vi "Dashboard Main.vi"() -> ()   [LabVIEW 2012]
uses:
  <vilib>/event_ctls.llb/eventvkey.ctl
  <vilib>/Utility/config.llb/Read Key (String).vi
  <vilib>/Utility/config.llb/Read Key (I32).vi
  <vilib>/Utility/config.llb/Write Key (String).vi
  <vilib>/Utility/config.llb/Write Key (I32).vi
  <vilib>/Utility/config.llb/NI_LVConfig.lvlib
panel:
  out "Mode":T1(ring)=enum."Auto Disabled"
  in  "Viewer":enum32{"Camera Image", "Variables"}(tab)
  out "Mbps":dbl format="%#.1g"
  in  "Enable":bool
  in  "DB Camera Config":bool
  out "Mbps":bool
  out "fps":dbl format="%#.1g"
  out "Image Error Message":string="Timeout in Camera Communications"
  out "Camera Image":T2(plugin-control)
  out "Camera Image 2":T2(plugin-control)
  in  "Camera Settings":T3={"Frame Rate"=15, "Compression"=30, "Size"=1} {"Frame Rate" scale=1.0..30.0; "Size" items=["640x480", "320x240", "160x120"]}
  out "Camera IP 2":string
  out "Camera IP":string
  out "fps 2":dbl format="%#.1g"
  out "Mbps 2":dbl format="%#.1g"
  in  "Enable 2":bool
  in  "FR":i32=15
  out "Tree":string(tree)
  in  "Dashboard Tab":enum32{"Operation", "Test", "Checklist"}(tab)
  in  "AutonRefresh":bool
  out "Autons":string[](array[string])
  in  "Selector":bool[](array[boolean])
  in  "Slider":dbl(slide) scale=0.0..100.0 scale format="%#_3g"
  in  "On/Off":bool caption="Solenoid"
  in  "Test Name":u16(ring) items=["Select the test to run...", "Example Test", "-------------------------------", "List of tests is built in robot code.", "Replace with your own automated tests."]
  in  "Test Tree":string(tree)
  in  "Motor":cluster{"Value":dbl, "Enable":bool} {"Value" scale=-1.0..1.0 scale format="%#_3g"}
  out "Progress":T4 {"Test Progress" scale=0.0..100.0}
  in  "Rev/Fwd":cluster{"Forward":bool, "Reverse":bool}
  in  "Ring":u16(ring) items=["Auto", "Fixed indoor", "Fixed outdoor 1", "Fixed outdoor 2", "Fixed fluorescent 1", "Fixed fluorescent 2", "Hold current"]
  in  "Listbox":i32(listbox)
  out "Robot IP":string
  out "Battery Value":dbl(slide) scale=0.0..14.0 scale format="%#_2e"
  out "Battery":sgl(graph)
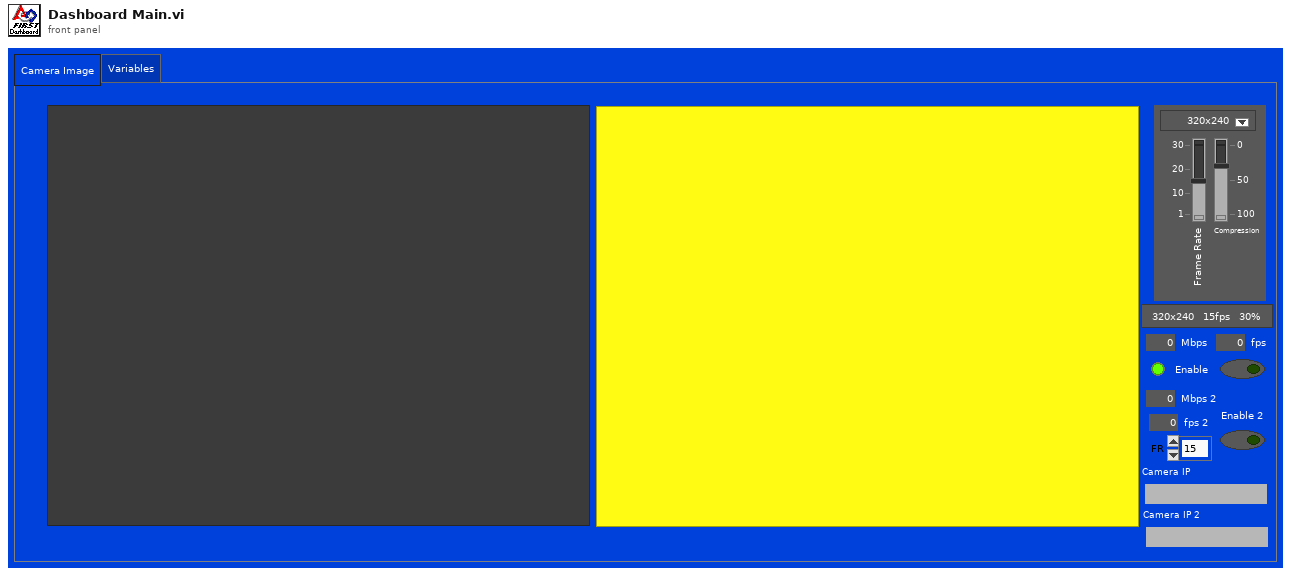
[diagram p1: front panel]
types:
  T1 = enum8{"Tele-Op Disabled", "Tele-Op Enabled", "Auto Disabled", "Auto Enabled", "Test Disabled", "Test Enabled", ""}
  T2 = typedef "IMAQ Image.ctl" = refnum<image>
  T3 = cluster{"Frame Rate":i32, "Compression":i32, "Size":u16}
  T4 = cluster{"Test Progress":u8, "Test Progress Text":string}
  T5 = typedef "Image Type" = u32
  T6 = cluster{"Competition mode":bool, "Robot Link":bool, "Autonomous":bool, "Enabled":bool, "E-Stop":bool, "Simulated":bool, "TestMode":bool, "Docked Window":bool}
  T7 = typedef "LVRectTypeDef.ctl" = cluster{"Left":i16, "Top":i16, "Right":i16, "Bottom":i16}
  T8 = typedef "NI_LVConfig.lvlib/Config Data RefNum.ctl" = refnum<k1>
  T9 = typedef "eventvkey.ctl" = enum16{"ASCII", "Enter", "Return", "Shift", "Ctrl", "Alt", "Cmd", "Opt", "Caps", "NumLock", "Clear", "Break", "Up", "Down", "Left", "Right", "Insert", "Delete", "Home", "End", "PageUp", "PageDown", "Escape", "Help", "Pause", "ScrollLock", "F1", "F2", "F3", "F4", "F5", "F6", "F7", "F8", "F9", "F10", "F11", "F12", "F13", "F14", "F15", "F16", "F17", "F18", "F19", "F20", "F21", "F22", "F23", "F24", "Play", "VolumeUp", "VolumeDown", "Mute", "Two Byte Char"}
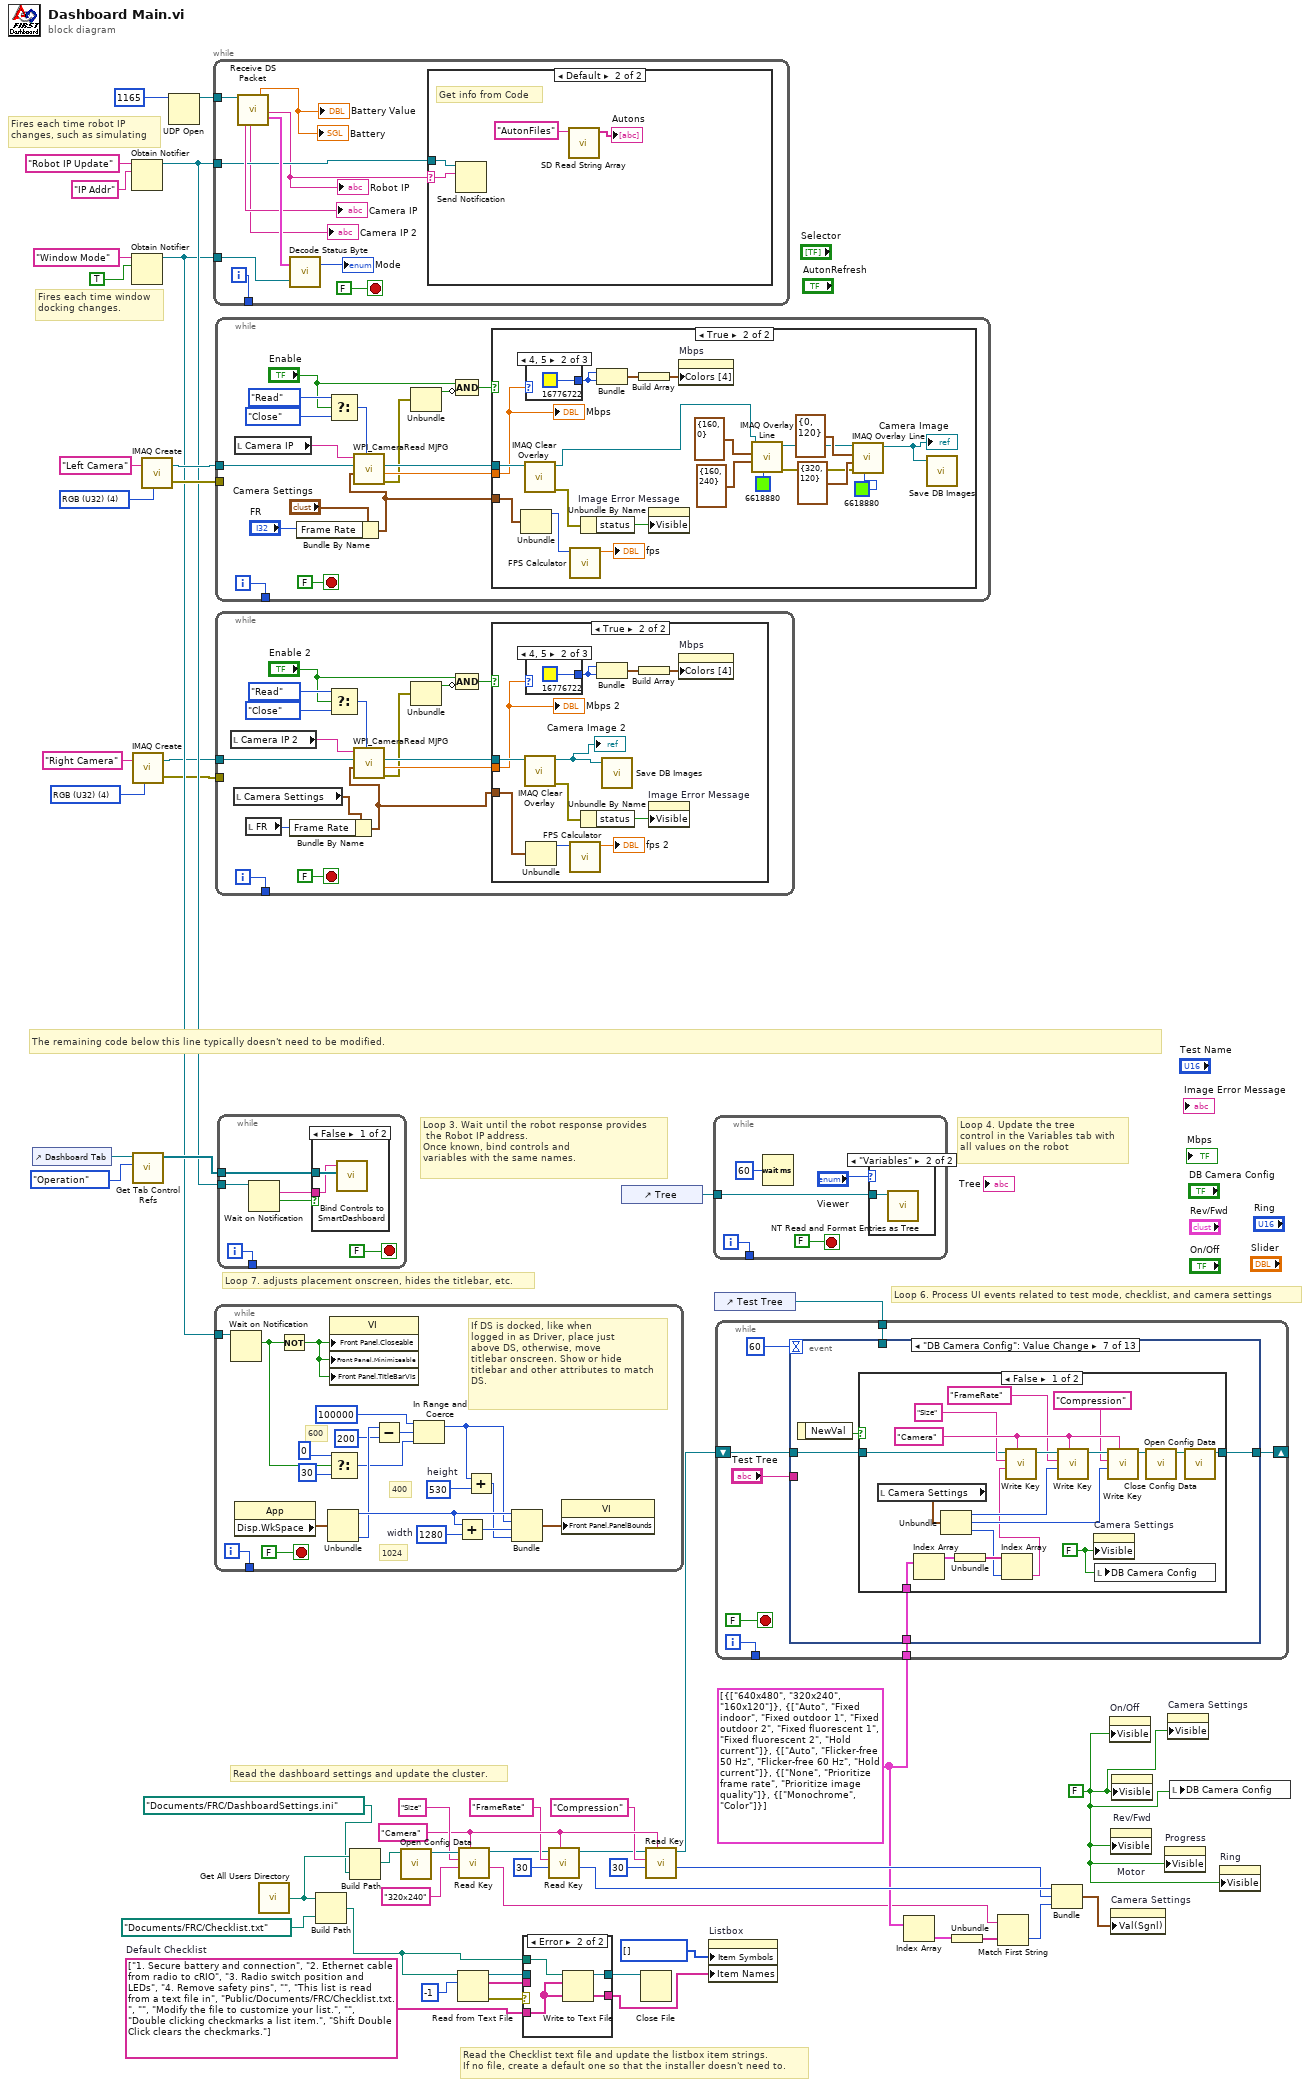
[diagram p0: block diagram]
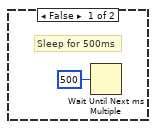
[diagram p2: hidden frame]
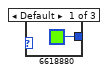
[diagram p3: hidden frame]
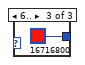
[diagram p4: hidden frame]
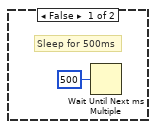
[diagram p6: hidden frame]
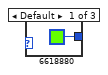
[diagram p7: hidden frame]
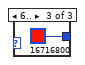
[diagram p8: hidden frame]
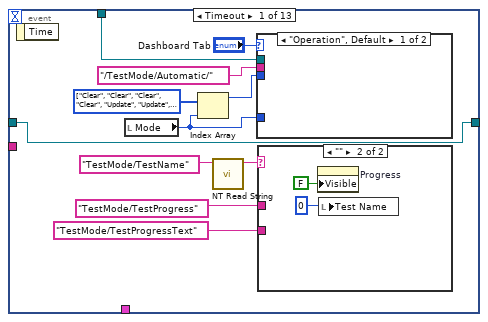
[diagram p10: hidden frame]
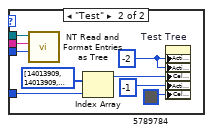
[diagram p11: hidden frame]
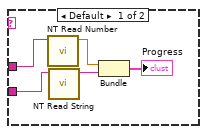
[diagram p12: hidden frame]
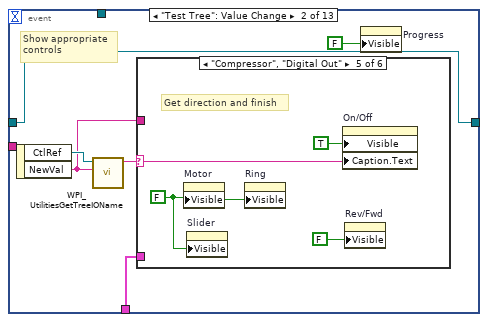
[diagram p13: hidden frame]
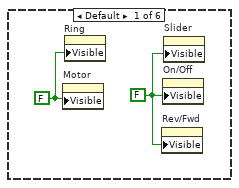
[diagram p14: hidden frame]
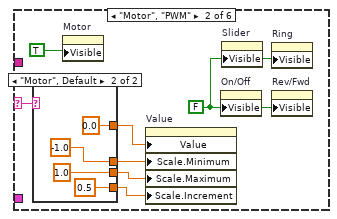
[diagram p15: hidden frame]
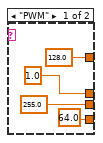
[diagram p16: hidden frame]
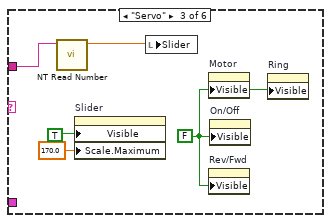
[diagram p17: hidden frame]
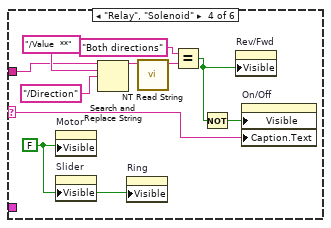
[diagram p18: hidden frame]
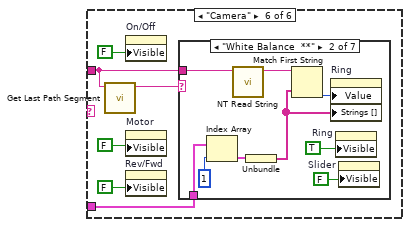
[diagram p19: hidden frame]
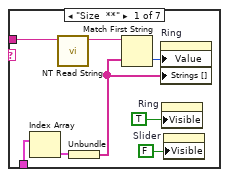
[diagram p20: hidden frame]
diagram:
  w3 = T5 4 items=["Grayscale (U8)", "Grayscale (I16)", "Grayscale (SGL)", "Complex (CSG)", "RGB (U32)", "HSL (U32)", "RGB (U64)"] ("Image Type")
  w25 = "Camera"
  w17 = cluster{string[]}[] [{["640x480", "320x240", "160x120"]}, {["Auto", "Fixed indoor", "Fixed outdoor 1", "Fixed outdoor 2", "Fixed fluorescent 1", "Fixed fluorescent 2", "Hold current"]}, {["Auto", "Flicker-free 50 Hz", "Flicker-free 60 Hz", "Hold current"]}, {["None", "Prioritize frame rate", "Prioritize image quality"]}, {["Monochrome", "Color"]}]
  w33 = string[] ["1. Secure battery and connection", "2. Ethernet cable from radio to cRIO", "3. Radio switch position and LEDs", "4. Remove safety pins", "", "This list is read from a text file in", "Public/Documents/FRC/Checklist.txt.", "", "Modify the file to customize your list.", "", "Double clicking checkmarks a list item.", "Shift Double Click clears the checkmarks."]  # Default Checklist
  w31 = FALSE ("Visible")
  w52 = T5 4 items=["Grayscale (U8)", "Grayscale (I16)", "Grayscale (SGL)", "Complex (CSG)", "RGB (U32)", "HSL (U32)", "RGB (U64)"] ("Image Type")
  # "Fires each time robot IP\nchanges, such as simulating"
  # "Fires each time window\ndocking changes."
  # "Read the Checklist text file and update the listbox item strings.\nIf no file, create a default one so that the installer doesn't need to."
  # "The remaining code below this line typically doesn't need to be modified."
  # "Loop 6. Process UI events related to test mode, checklist, and camera settings"
  # "Read the dashboard settings and update the cluster."
  # "Loop 4. Update the tree\ncontrol in the Variables tab with\nall values on the robot"
  # "Loop 3. Wait until the robot response provides\n the Robot IP address.\nOnce known, bind controls and\nvariables with the same names."
  # "Loop 7. adjusts placement onscreen, hides the titlebar, etc."
  n1 = control-ref of="Dashboard Tab"() -> (w47:refnum<vi>)
  n2 = Obtain Notifier(name (unnamed)="Robot IP Update", notification data type="IP Addr" ("name (unnamed)")) -> (notifier out=w44:refnum<notifier>)  [unwired: 2 in, 2 out]
  n3 = Obtain Notifier(name (unnamed)="Window Mode", notification data type=TRUE) -> (notifier out=w37:refnum<notifier>)  [unwired: 2 in, 2 out]
  n4 = call "IMAQ Create"("Image Name"="Right Camera", "Image Type"=w3) -> ("New Image"=w2:T2, "error out"=w1:errorcluster)  [unwired: 2 in, 1 out]
  n5 = call <vilib>:"Get Tab Control Refs.vi"("Page Index"=enum32{"Operation", "Test"}."Operation" ("Dashboard Tab"), "TabControl in"=w47) -> ("ControlsOnPage"=w48:refnum<vi>[])  [unwired: 9 in]
  n6 = call "IMAQ Create"("Image Name"="Left Camera", "Image Type"=w52) -> ("New Image"=w50:T2, "error out"=w49:errorcluster)  [unwired: 2 in, 1 out]
  n7 = UDP Open(11:u16 1165 ("port")) -> (port=w53:refnum<k16>)  [unwired: 2 in, 4 out]
  n8 = while {
    tunnel: w53 -> [w63]
    tunnel: w44 -> [w57]
    tunnel: w37 -> [w61]
    tunnel: [w58] -> _
    i -> [w58]
    stop <- FALSE stop-if-true
    n9 = call "Receive DS Packet.vi"("Recv Socket"=w63) -> ("Camera IP Address"=→"Camera IP":string, "Camera IP Address 2"=→"Camera IP 2":string, "Battery"=→"Battery" →"Battery Value":sgl, "Robot IP Address"=w56:string, "Status"=w64:T6)  [unwired: 8 in, 6 out]
    "Robot IP" <- w56
    n10 = call "Decode Status Byte.vi"("Window Mode Notifier"=w61, "Status"=w64) -> ("Mode"=→"Mode":T1)  [unwired: 1 out]
    n11 = case shown="Default" w56 {
      selector: w56 -> [_ w68]
      tunnel: w57 -> [_ w69]
      frame "0.0.0.0" {
        # "Robot not responding, don't poll the variables"
      }
      frame Default {
        # "Get info from Code"
        n12 = Send Notification(notification=w68, notifier=w69) -> ()  [unwired: 1 in, 2 out]
        n13 = call <vilib>:"SD Read String Array.vi"("Name"="AutonFiles") -> ("String Array"=→"Autons":string[])  [unwired: 9 in, 1 out]
      }
    }
  }
  n14 = while {
    tunnel: w37 -> [w88]
    tunnel: [w86] -> _
    i -> [w86]
    stop <- FALSE stop-if-true
    w78 = 1280  # width
    w81 = 530  # height
    # "600"
    # "1024"
    # "400"
    # "If DS is docked, like when\nlogged in as Driver, place just\nabove DS, otherwise, move\ntitlebar onscreen. Show or hide\ntitlebar and other attributes to match\nDS."
    n15 = Wait on Notification(notifier=w88) -> (notification=w73:bool)  [unwired: 3 in, 3 out]
    n16 = property class="App"() -> ("Disp.WkSpace"=w84:T7)  [unwired: 2 in, 2 out]
    n17 = Not(x=w73) -> (.not. x?=w87:bool)
    n18 = Unbundle(w84) -> ("Left"=w82:i16, "Bottom"=w79:i16)  [unwired: 2 out]
    n19 = Select(t=0, s=w73, f=30) -> (s? t:f=w72:i32)
    n20 = property class="VI"("Front Panel.Closeable"=w87, "Front Panel.Minimizeable"=w87, "Front Panel.TitleBarVis"=w87) -> ()  [unwired: 2 in, 2 out]
    n21 = Subtract(x=w79, y=200) -> (x-y=w76:i32)
    n22 = In Range and Coerce(upper limit=100000, x=w76, lower limit=w72) -> (coerced(x)=w70:i32)  [unwired: 1 out]
    n23 = Add(x=w82, y=w78) -> (x+y=w83:i32)
    n24 = Add(x=w70, y=w81) -> (x+y=w80:i32)
    n25 = Bundle("Left"=w82, w70, w83, w80) -> (w85:cluster{"Left":i16, i32, i32, i32})  [unwired: 1 out]
    n26 = property class="VI"("Front Panel.PanelBounds"=w85) -> ()  [unwired: 2 in, 2 out]
  }
  n27 = while {
    tunnel: w50 -> [w102]
    tunnel: w49 -> [_]
    tunnel: [w104] -> _
    i -> [w104]
    stop <- FALSE stop-if-true
    n28 = local read "Camera IP"() -> (w103:string)
    n29 = Bundle By Name(cluster="Camera Settings", "Frame Rate"="FR") -> (w90:T3)
    n30 = Select(t=enum16{"Read", "Reopen", "Close"}."Read" ("Operation"), s="Enable", f=enum16{"Read", "Reopen", "Close"}."Close" ("Operation")) -> (s? t:f=w97:enum16{"Read", "Reopen", "Close"})
    n31 = call <vilib>:"WPI_CameraRead MJPG.vi"("Operation"=w97, "Camera Settings"=w90, "Image"=w102, "address"=w103) -> ("error out"=w96:errorcluster, "Bandwidth (kbps)"=w100:dbl, "Image Out"=w101:T2)  [unwired: 5 in]
    n32 = Unbundle(w96) -> ("status"=w94:bool)  [unwired: 2 out]
    n33 = Compound Arithmetic op=AND("Enable", invert w94) -> (w93:bool)
    n34 = case shown="True" w93 {
      tunnel: w90 -> [_ w118]
      tunnel: w101 -> [_ w121]
      tunnel: w100 -> [_ w120]
      frame False {
        # "Sleep for 500ms"
        n35 = Wait Until Next ms Multiple(millisecond multiple=u32 500) -> ()  [unwired: 1 out]
      }
      frame True {
        n36 = Unbundle(w118) -> ("Frame Rate"=w108:i32)  [unwired: 2 out]
        n37 = call "IMAQ Clear Overlay"("Image"=w121) -> ("error out"=w125:errorcluster, "Image Out"=w110:T2)  [unwired: 2 in, 7 out]
        n38 = case shown="4, 5" w120 {
          tunnel: [u32 6618880 ("Color Box") u32 16776722 ("Color Box") u32 16716800 ("Color Box")] -> w122
          frame Default {
          }
          frame 4, 5 {
          }
          frame 6.. {
          }
        }
        n39 = call "FPS Calculator.vi"("Average Count"=w108) -> ("fps"=→"fps":dbl)  [unwired: 10 in]
        n40 = Unbundle By Name(w125) -> ("status"=w126:bool)
        n41 = Bundle("Color Box"=w122, "Color Box"=w122) -> (w124:cluster{"Color Box":u32, "Color Box":u32})  [unwired: 1 out]
        n42 = Build Array(w124) -> (w123:cluster{"Color Box":u32, "Color Box":u32}[])
        n43 = property on="Image Error Message" class="Str"("Visible"=w126) -> ()  [unwired: 2 in, 2 out]
        n44 = property on="Mbps" class="Bool (strict)"("Colors [4]"=w123) -> ()  [unwired: 2 in, 2 out]
        n45 = call "IMAQ Overlay Line"("Color"=u32 6618880, "End Point"=cluster{"X":i32, "Y":i32} {"X"=160, "Y"=240}, "Start Point"=cluster{"X":i32, "Y":i32} {"X"=160, "Y"=0}, "Image"=w110) -> ("error out"=w115:errorcluster, "Image Out"=w114:T2)  [unwired: 6 in]
        n46 = call "IMAQ Overlay Line"("Color"=u32 6618880, "error in (no error)"=w115, "End Point"=cluster{"X":i32, "Y":i32} {"X"=320, "Y"=120}, "Start Point"=cluster{"X":i32, "Y":i32} {"X"=0, "Y"=120}, "Image"=w114) -> ("Image Out"=w109:T2)  [unwired: 5 in, 1 out]
        "Camera Image" <- w109
        n47 = call "Save DB Images.vi"("Image"=w109) -> ()  [unwired: 2 in, 1 out]
        "Mbps" <- w120
      }
    }
  }
  n48 = while {
    tunnel: w2 -> [w142]
    tunnel: [w144] -> _
    tunnel: w1 -> [_]
    i -> [w144]
    stop <- FALSE stop-if-true
    n49 = local read "Camera IP 2"() -> (w143:string)
    n50 = local read "Camera Settings"() -> (w131:T3)
    n51 = local read "FR"() -> (w132:i32)
    n52 = Bundle By Name(cluster=w131, "Frame Rate"=w132) -> (w130:T3)
    n53 = Select(t=enum16{"Read", "Reopen", "Close"}."Read" ("Operation"), s="Enable 2", f=enum16{"Read", "Reopen", "Close"}."Close" ("Operation")) -> (s? t:f=w137:enum16{"Read", "Reopen", "Close"})
    n54 = call <vilib>:"WPI_CameraRead MJPG.vi"("Operation"=w137, "Camera Settings"=w130, "Image"=w142, "address"=w143) -> ("error out"=w136:errorcluster, "Bandwidth (kbps)"=w140:dbl, "Image Out"=w141:T2)  [unwired: 5 in]
    n55 = Unbundle(w136) -> ("status"=w134:bool)  [unwired: 2 out]
    n56 = Compound Arithmetic op=AND("Enable 2", invert w134) -> (w133:bool)
    n57 = case shown="True" w133 {
      tunnel: w130 -> [_ w149]
      tunnel: w141 -> [_ w152]
      tunnel: w140 -> [_ w151]
      frame False {
        # "Sleep for 500ms"
        n58 = Wait Until Next ms Multiple(millisecond multiple=u32 500) -> ()  [unwired: 1 out]
      }
      frame True {
        n59 = call "IMAQ Clear Overlay"("Image"=w152) -> ("error out"=w156:errorcluster, "Image Out"=w147:T2)  [unwired: 2 in, 7 out]
        "Camera Image 2" <- w147
        n60 = case shown="4, 5" w151 {
          tunnel: [u32 6618880 ("Color Box") u32 16776722 ("Color Box") u32 16716800 ("Color Box")] -> w153
          frame Default {
          }
          frame 4, 5 {
          }
          frame 6.. {
          }
        }
        n61 = Unbundle(w149) -> ("Frame Rate"=w148:i32)  [unwired: 2 out]
        n62 = call "FPS Calculator.vi"("Average Count"=w148) -> ("fps"=→"fps 2":dbl)  [unwired: 10 in]
        n63 = Unbundle By Name(w156) -> ("status"=w157:bool)
        n64 = Bundle("Color Box"=w153, "Color Box"=w153) -> (w155:cluster{"Color Box":u32, "Color Box":u32})  [unwired: 1 out]
        n65 = call "Save DB Images.vi"("Image"=w147) -> ()  [unwired: 2 in, 1 out]
        n66 = Build Array(w155) -> (w154:cluster{"Color Box":u32, "Color Box":u32}[])
        n67 = property on="Image Error Message" class="Str"("Visible"=w157) -> ()  [unwired: 2 in, 2 out]
        n68 = property on="Mbps" class="Bool (strict)"("Colors [4]"=w154) -> ()  [unwired: 2 in, 2 out]
        "Mbps 2" <- w151
      }
    }
  }
  n69 = while {
    tunnel: w48 -> [w166]
    tunnel: w44 -> [w163]
    tunnel: [w161] -> _
    i -> [w161]
    stop <- FALSE stop-if-true
    n70 = Wait on Notification(notifier=w163) -> (notification=w162:string, timed out?=w164:bool)  [unwired: 3 in, 2 out]
    n71 = case shown="False" w164 {
      tunnel: w166 -> [w168 _]
      tunnel: w162 -> [w167 _]
      frame False {
        n72 = call <vilib>:"Bind Controls to SmartDashboard.vi"("Bound Control Refs"=w168, "Server IP Address"=w167) -> ()  [unwired: 10 in]
      }
      frame True {
      }
    }
  }
  n73 = call "Get All Users Directory.vi"() -> ("All User Path"=w30:path)
  n74 = Build Path(base path=w30, name or relative path=path "Documents/FRC/Checklist.txt") -> (appended path=w34:path)
  n75 = Build Path(base path=w30, name or relative path=path "Documents/FRC/DashboardSettings.ini") -> (appended path=w29:path)
  n76 = call <vilib>:"Open Config Data.vi"("configuration file path"=w29) -> ("refnum"=w28:T8)  [unwired: 8 in, 2 out]
  n77 = Read from Text File(file (use dialog)=w34, count=-1 ("timeout ms (25000)")) -> (refnum out=w12:refnum<file>, text=w35:string[], error out=w36:errorcluster)  [unwired: 2 in, 1 out]
  n78 = call-poly <vilib>:"Read Key.vi"("section"=w25, "default value"="320x240", "key"="Size", "refnum"=w28) -> ("value"=w15:string, "refnum out"=w10:T8)  [unwired: 2 in, 4 out]
  n79 = case shown="Error" w36 {
    tunnel: w35 -> [w170 _]
    tunnel: [w170 w172] -> w32
    tunnel: w33 -> [_ w172]
    tunnel: w34 -> [_ w173]
    tunnel: [w169 w171] -> w11
    tunnel: w12 -> [w169 _]
    frame No Error {
    }
    frame Error {
      n80 = Write to Text File(file (use dialog)=w173, text=w172) -> (refnum out=w171:refnum<file>)  [unwired: 2 in, 2 out]
    }
  }
  n81 = call-poly <vilib>:"Read Key.vi"("section"=w25, "default value"=30, "key"="FrameRate", "refnum"=w10) -> ("value"=w20:i32, "refnum out"=w9:T8)  [unwired: 1 in, 5 out]
  n82 = control-ref of="Tree"() -> (w6:refnum<vi>)
  n83 = Close File(refnum=w11) -> ()  [unwired: 1 in, 2 out]
  n84 = call-poly <vilib>:"Read Key.vi"("section"=w25, "default value"=30, "key"="Compression", "refnum"=w9) -> ("value"=w19:i32, "refnum out"=w7:T8)  [unwired: 1 in, 5 out]
  n85 = property on="Listbox" class="LstBox (strict)"("Item Symbols"=i32[] [], "Item Names"=w32) -> ()  [unwired: 2 in, 2 out]
  n86 = while {
    tunnel: [w175] -> _
    tunnel: w6 -> [w174]
    i -> [w175]
    stop <- FALSE stop-if-true
    n87 = Wait (ms)(milliseconds to wait=u32 60) -> ()  [unwired: 1 out]
    n88 = case shown="\"Variables\"" "Viewer" {
      tunnel: w174 -> [_ w179]
      frame Default {
      }
      frame "Variables" {
        n89 = call <vilib>:"NT Read and Format Entries as Tree.vi"("Tree Refnum"=w179) -> ()  [unwired: 9 in, 2 out]
      }
    }
  }
  n90 = control-ref of="Test Tree"() -> (w5:refnum<vi>)
  n91 = while {
    tunnel: w17 -> [w184]
    shift-right: [w183] -> _
    shift-left: w7 -> [w182]
    tunnel: [w181] -> _
    tunnel: w5 -> [w180]
    i -> [w181]
    stop <- FALSE stop-if-true
    n92 = event shown="[6] \"DB Camera Config\": Value Change" {
      selector: _ -> [_ _ _ _ _ _ _ _ _ _ _ _ _]
      dyn-events: _ -> [_ _ _ _ _ _ _ _ _ _ _ _ _]
      timeout: u32 60 ("milliseconds to wait") -> [_ _ _ _ _ _ _ _ _ _ _ _ _]
      tunnel: w180 -> [w194 _ _ _ _ _ _ _ _ _ _ _ _]
      tunnel: "Test Tree" -> [_ _ _ _ _ _ _ _ w388 w396 w398 w402 w410]
      tunnel: w184 -> [_ w216 _ _ _ _ w352 w382 _ _ _ _ _]
      tunnel: [w188 w215 _ w318 w326 w338 w351 w375 w387 w394 w397 w401 w409] -> w183
      tunnel: w182 -> [w188 w215 _ w318 w326 w338 w350 w375 w387 w394 w397 w401 w409]
      event Timeout {
        w193 = enum16{"Update", "Clear"}[] [enum."Clear", enum."Clear", enum."Clear", enum."Clear", enum."Update", enum."Update", enum."Clear"] items=["Update", "Clear"]
        n93 = event-data() -> ()  [unwired: 1 in, 1 out]
        n94 = local read "Mode"() -> (w191:T1)
        n95 = Index Array(array=w193, index=w191) -> (element=w192:enum16{"Update", "Clear"})
        n96 = call <vilib>:"NT Read String.vi"("Name"="TestMode/TestName") -> ("String"=w197:string)  [unwired: 9 in, 1 out]
        n97 = case shown="\"Operation\", Default" "Dashboard Tab" {
          tunnel: w194 -> [_ w207]
          tunnel: "/TestMode/Automatic/" ("Name Pattern") -> [_ w206]
          tunnel: w192 -> [_ w205]
          tunnel: w191 -> [_ w203]
          frame "Operation", Default {
          }
          frame "Test" {
            w202 = -2 ("Active Item:Row Number")
            n98 = call <vilib>:"NT Read and Format Entries as Tree.vi"("Operation"=w205, "Name Pattern"=w206, "Tree Refnum"=w207) -> ()  [unwired: 7 in, 2 out]
            n99 = Index Array(array=u32[] [14013909, 14013909, 14013909, 14013909, 14013909, 16777215, 14013909], index=w203) -> (element=w201:u32)
            n100 = property on="Test Tree" class="Tree (strict)"("Active Item Row Number"=w202, "ActiveColNum"=w202, "CellBG"=w201, "Active Item Row Number"=-1 ("Active Item:Row Number"), "CellBG"=u32 5789784 ("Color Box")) -> ()  [unwired: 2 in, 2 out]
          }
        }
        n101 = case shown="\"\"" w197 {
          tunnel: "TestMode/TestProgress" ("Name") -> [w209 _]
          tunnel: "TestMode/TestProgressText" ("Name") -> [w208 _]
          frame Default {
            n102 = call <vilib>:"NT Read Number.vi"("Name"=w209) -> ("Numeric"=w210:dbl)  [unwired: 9 in, 1 out]
            n103 = call <vilib>:"NT Read String.vi"("Name"=w208) -> ("String"=w211:string)  [unwired: 9 in, 1 out]
            n104 = Bundle("Numeric"=w210, "String"=w211) -> (→"Progress":cluster{"Numeric":dbl, "String":string})  [unwired: 1 in]
          }
          frame "" {
            n105 = property on="Progress" class="Clust (strict)"("Visible"=FALSE) -> ()  [unwired: 2 in, 2 out]
            n106 = local write "Test Name"(u16 0) -> ()
          }
        }
      }
      event "Test Tree": Value Change {
        # "Show appropriate\ncontrols"
        n107 = event-data() -> ("CtlRef"=w219:refnum<vi>, "NewVal"=w217:string)  [unwired: 1 in]
        n108 = call <vilib>:"WPI_UtilitiesGetTreeIOName.vi"("NewVal"=w217, "TreeControl in"=w219) -> ("I/O Name"=w220:string)  [unwired: 9 in]
        n109 = case shown="\"Compressor\", \"Digital Out\"" w220 {
          selector: w220 -> [_ w227 _ w245 w254 _]
          tunnel: w217 -> [_ _ w242 w244 _ w261]
          tunnel: w216 -> [_ _ _ _ _ w260]
          frame Default {
            w222 = FALSE ("Visible")
            w221 = FALSE ("Visible")
            n110 = property on="Motor" class="Clust (strict)"("Visible"=w221) -> ()  [unwired: 2 in, 2 out]
            n111 = property on="Ring" class="Ring (strict)"("Visible"=w221) -> ()  [unwired: 2 in, 2 out]
            n112 = property on="Rev/Fwd" class="Clust (strict)"("Visible"=w222) -> ()  [unwired: 2 in, 2 out]
            n113 = property on="On/Off" class="Bool (strict)"("Visible"=w222) -> ()  [unwired: 2 in, 2 out]
            n114 = property on="Slider" class="Slide (strict)"("Visible"=w222) -> ()  [unwired: 2 in, 2 out]
          }
          frame "Motor", "PWM" {
            w228 = FALSE ("Visible")
            n115 = case shown="\"Motor\", Default" w227 {
              tunnel: [1.0 ("Value") -1.0 ("Value")] -> w226
              tunnel: [255.0 ("Value") 1.0 ("Value")] -> w225
              tunnel: [128.0 ("Value") 0.0 ("Value")] -> w224
              tunnel: [64.0 ("Value") 0.5 ("Value")] -> w223
              frame "PWM" {
              }
              frame "Motor", Default {
              }
            }
            n116 = property on="Motor" class="Clust (strict)"("Visible"=TRUE) -> ()  [unwired: 2 in, 2 out]
            n117 = property on="Value" class="Slide (strict)"("Value"=w224, "Scale.Minimum"=w226, "Scale.Maximum"=w225, "Scale.Increment"=w223) -> ()  [unwired: 2 in, 2 out]
            n118 = property on="On/Off" class="Bool (strict)"("Visible"=w228) -> ()  [unwired: 2 in, 2 out]
            n119 = property on="Slider" class="Slide (strict)"("Visible"=w228) -> ()  [unwired: 2 in, 2 out]
            n120 = property on="Ring" class="Ring (strict)"("Visible"=w228) -> ()  [unwired: 2 in, 2 out]
            n121 = property on="Rev/Fwd" class="Clust (strict)"("Visible"=w228) -> ()  [unwired: 2 in, 2 out]
          }
          frame "Servo" {
            w240 = FALSE ("Visible")
            n122 = call <vilib>:"NT Read Number.vi"("Name"=w242) -> ("Numeric"=w241:dbl)  [unwired: 9 in, 1 out]
            n123 = property on="Slider" class="Slide (strict)"("Visible"=TRUE, "Scale.Maximum"=170.0 ("Scale.Range:Maximum")) -> ()  [unwired: 2 in, 2 out]
            n124 = local write "Slider"(w241) -> ()
            n125 = property on="Motor" class="Clust (strict)"("Visible"=w240) -> ()  [unwired: 2 in, 2 out]
            n126 = property on="Rev/Fwd" class="Clust (strict)"("Visible"=w240) -> ()  [unwired: 2 in, 2 out]
            n127 = property on="On/Off" class="Bool (strict)"("Visible"=w240) -> ()  [unwired: 2 in, 2 out]
            n128 = property on="Ring" class="Ring (strict)"("Visible"=w240) -> ()  [unwired: 2 in, 2 out]
          }
          frame "Relay", "Solenoid" {
            w243 = FALSE ("Visible")
            n129 = property on="Motor" class="Clust (strict)"("Visible"=w243) -> ()  [unwired: 2 in, 2 out]
            n130 = property on="Slider" class="Slide (strict)"("Visible"=w243) -> ()  [unwired: 2 in, 2 out]
            n131 = Search and Replace String(input string=w244, search string="/Value  **", replace string="/Direction") -> (result string=w250:string)  [unwired: 5 in, 3 out]
            n132 = property on="Ring" class="Ring (strict)"("Visible"=w243) -> ()  [unwired: 2 in, 2 out]
            n133 = call <vilib>:"NT Read String.vi"("Name"=w250) -> ("String"=w248:string)  [unwired: 9 in, 1 out]
            n134 = Equal?(x="Both directions", y=w248) -> (x = y?=w246:bool)
            n135 = Not(x=w246) -> (.not. x?=w247:bool)
            n136 = property on="Rev/Fwd" class="Clust (strict)"("Visible"=w246) -> ()  [unwired: 2 in, 2 out]
            n137 = property on="On/Off" class="Bool (strict)"("Visible"=w247, "Caption.Text"=w245) -> ()  [unwired: 2 in, 2 out]
          }
          frame "Compressor", "Digital Out" {
            w253 = FALSE ("Visible")
            # "Get direction and finish"
            n138 = property on="Motor" class="Clust (strict)"("Visible"=w253) -> ()  [unwired: 2 in, 2 out]
            n139 = property on="Slider" class="Slide (strict)"("Visible"=w253) -> ()  [unwired: 2 in, 2 out]
            n140 = property on="Ring" class="Ring (strict)"("Visible"=w253) -> ()  [unwired: 2 in, 2 out]
            n141 = property on="On/Off" class="Bool (strict)"("Visible"=TRUE, "Caption.Text"=w254) -> ()  [unwired: 2 in, 2 out]
            n142 = property on="Rev/Fwd" class="Clust (strict)"("Visible"=FALSE) -> ()  [unwired: 2 in, 2 out]
          }
          frame "Camera" {
            n143 = call <vilib>:"Get Last Path Segment.vi"("String in"=w261) -> ("String out"=w262:string)  [unwired: 10 in]
            n144 = property on="On/Off" class="Bool (strict)"("Visible"=FALSE) -> ()  [unwired: 2 in, 2 out]
            n145 = property on="Motor" class="Clust (strict)"("Visible"=FALSE) -> ()  [unwired: 2 in, 2 out]
            n146 = property on="Rev/Fwd" class="Clust (strict)"("Visible"=FALSE) -> ()  [unwired: 2 in, 2 out]
            n147 = case shown="\"White Balance  **\"" w262 {
              tunnel: w261 -> [w268 w277 w286 w295 w304 _ w310]
              tunnel: w260 -> [w266 w274 w283 w292 w301 _ _]
              frame "Size  **" {
                n148 = Index Array(array=w266) -> (element=w265:cluster{string[]})  [unwired: 1 in]
                n149 = call <vilib>:"NT Read String.vi"("Name"=w268) -> ("String"=w267:string)  [unwired: 9 in, 1 out]
                n150 = Unbundle(w265) -> (w263:string[])
                n151 = Match First String(2:w263, 3:w267) -> (0:w264:i32)  [unwired: 1 out]
                n152 = property on="Ring" class="Ring (strict)"("Value"=w264, "Strings []"=w263) -> ()  [unwired: 2 in, 2 out]
                n153 = property on="Ring" class="Ring (strict)"("Visible"=TRUE) -> ()  [unwired: 2 in, 2 out]
                n154 = property on="Slider" class="Slide (strict)"("Visible"=FALSE) -> ()  [unwired: 2 in, 2 out]
              }
              frame "White Balance  **" {
                n155 = Index Array(array=w274, index=1) -> (element=w275:cluster{string[]})
                n156 = call <vilib>:"NT Read String.vi"("Name"=w277) -> ("String"=w276:string)  [unwired: 9 in, 1 out]
                n157 = Unbundle(w275) -> (w272:string[])
                n158 = Match First String(2:w272, 3:w276) -> (0:w271:i32)  [unwired: 1 out]
                n159 = property on="Ring" class="Ring (strict)"("Value"=w271, "Strings []"=w272) -> ()  [unwired: 2 in, 2 out]
                n160 = property on="Ring" class="Ring (strict)"("Visible"=TRUE) -> ()  [unwired: 2 in, 2 out]
                n161 = property on="Slider" class="Slide (strict)"("Visible"=FALSE) -> ()  [unwired: 2 in, 2 out]
              }
              frame "Exposure  **" {
                n162 = Index Array(array=w283, index=2) -> (element=w284:cluster{string[]})
                n163 = call <vilib>:"NT Read String.vi"("Name"=w286) -> ("String"=w285:string)  [unwired: 9 in, 1 out]
                n164 = Unbundle(w284) -> (w280:string[])
                n165 = Match First String(2:w280, 3:w285) -> (0:w281:i32)  [unwired: 1 out]
                n166 = property on="Ring" class="Ring (strict)"("Value"=w281, "Strings []"=w280) -> ()  [unwired: 2 in, 2 out]
                n167 = property on="Ring" class="Ring (strict)"("Visible"=TRUE) -> ()  [unwired: 2 in, 2 out]
                n168 = property on="Slider" class="Slide (strict)"("Visible"=FALSE) -> ()  [unwired: 2 in, 2 out]
              }
              frame "Exposure Priority  **" {
                n169 = Index Array(array=w292, index=3) -> (element=w293:cluster{string[]})
                n170 = call <vilib>:"NT Read String.vi"("Name"=w295) -> ("String"=w294:string)  [unwired: 9 in, 1 out]
                n171 = Unbundle(w293) -> (w289:string[])
                n172 = Match First String(2:w289, 3:w294) -> (0:w290:i32)  [unwired: 1 out]
                n173 = property on="Ring" class="Ring (strict)"("Value"=w290, "Strings []"=w289) -> ()  [unwired: 2 in, 2 out]
                n174 = property on="Ring" class="Ring (strict)"("Visible"=TRUE) -> ()  [unwired: 2 in, 2 out]
                n175 = property on="Slider" class="Slide (strict)"("Visible"=FALSE) -> ()  [unwired: 2 in, 2 out]
              }
              frame "Color Enable  **" {
                n176 = Index Array(array=w301, index=4) -> (element=w302:cluster{string[]})
                n177 = call <vilib>:"NT Read String.vi"("Name"=w304) -> ("String"=w303:string)  [unwired: 9 in, 1 out]
                n178 = Unbundle(w302) -> (w298:string[])
                n179 = Match First String(2:w298, 3:w303) -> (0:w299:i32)  [unwired: 1 out]
                n180 = property on="Ring" class="Ring (strict)"("Value"=w299, "Strings []"=w298) -> ()  [unwired: 2 in, 2 out]
                n181 = property on="Ring" class="Ring (strict)"("Visible"=TRUE) -> ()  [unwired: 2 in, 2 out]
                n182 = property on="Slider" class="Slide (strict)"("Visible"=FALSE) -> ()  [unwired: 2 in, 2 out]
              }
              frame Default {
                n183 = property on="Ring" class="Ring (strict)"("Visible"=FALSE) -> ()  [unwired: 2 in, 2 out]
                n184 = property on="Slider" class="Slide (strict)"("Visible"=FALSE) -> ()  [unwired: 2 in, 2 out]
              }
              frame "Brightness  **", "Color Level  **", "Compression  **", "FPS  **", "Sharpness  **" {
                n185 = call <vilib>:"NT Read Number.vi"("Name"=w310) -> ("Numeric"=w309:dbl)  [unwired: 9 in, 1 out]
                n186 = local write "Slider"(w309) -> ()
                n187 = property on="Slider" class="Slide (strict)"("Visible"=TRUE, "Scale.Maximum"=100.0 ("Scale.Range:Maximum")) -> ()  [unwired: 2 in, 2 out]
                n188 = property on="Ring" class="Ring (strict)"("Visible"=FALSE) -> ()  [unwired: 2 in, 2 out]
              }
            }
          }
        }
        n189 = property on="Progress" class="Clust (strict)"("Visible"=FALSE) -> ()  [unwired: 2 in, 2 out]
      }
      event "Test Name": Mouse Enter {
        # "Populate the ring with the list of tests"
        n190 = event-data() -> ()  [unwired: 1 in, 1 out]
        n191 = call <vilib>:"NT Read String Array.vi"("Name"="TestMode/TestList") -> ("String Array"=w317:string[])  [unwired: 9 in, 1 out]
        n192 = Build Array (concatenate)("Select the test to run...", w317) -> (w316:string[])
        n193 = property on="Test Name" class="Ring (strict)"("Strings []"=w316) -> ()  [unwired: 2 in, 2 out]
      }
      event "Test Name": Value Change {
        w319 = FALSE ("Visible")
        # "Tell the robot the test name to run"
        n194 = event-data() -> ("NewVal"=w323:u16)  [unwired: 1 in]
        n195 = property on="Test Name" class="Ring (strict)"() -> ("Strings []"=w324:string[])  [unwired: 2 in, 2 out]
        n196 = local write "Progress"(T4 {"Test Progress"=0, "Test Progress Text"=""} ("Progress")) -> ()
        n197 = Index Array(array=w324, index=w323) -> (element=w322:string)
        n198 = call <vilib>:"NT Write String.vi"("String"=w322, "Name"="TestMode/TestName") -> ()  [unwired: 9 in, 1 out]
        n199 = property on="Progress" class="Clust (strict)"("Visible"=TRUE) -> ()  [unwired: 2 in, 2 out]
        n200 = property on="Motor" class="Clust (strict)"("Visible"=w319) -> ()  [unwired: 2 in, 2 out]
        n201 = property on="Slider" class="Slide (strict)"("Visible"=w319) -> ()  [unwired: 2 in, 2 out]
        n202 = property on="On/Off" class="Bool (strict)"("Visible"=w319) -> ()  [unwired: 2 in, 2 out]
        n203 = property on="Rev/Fwd" class="Clust (strict)"("Visible"=w319) -> ()  [unwired: 2 in, 2 out]
        n204 = property on="Ring" class="Ring (strict)"("Visible"=w319) -> ()  [unwired: 2 in, 2 out]
      }
      event "Listbox": Double Click {
        n205 = event-data() -> ("PlatMods.Shift"=w327:bool, "Row"=w329:i32)  [unwired: 1 in]
        n206 = case shown="False" w327 {
          tunnel: w329 -> [w333 _]
          tunnel: 1 -> [w332 _]
          frame False {
            n207 = property on="Listbox" class="LstBox (strict)"() -> ("Item Symbols"=w331:i32[])  [unwired: 2 in, 2 out]
            n208 = Replace Array Subset(array=w331, new element=w332, index=w333) -> (w330:i32[])
            n209 = property on="Listbox" class="LstBox (strict)"("Item Symbols"=w330) -> ()  [unwired: 2 in, 2 out]
          }
          frame True {
            w334 = 0 ("Top Row")
            n210 = property on="Listbox" class="LstBox (strict)"() -> ("Number of Rows"=w336:u32)  [unwired: 2 in, 2 out]
            n211 = Initialize Array(0, w336) -> (w335:i32[])
            n212 = property on="Listbox" class="LstBox (strict)"("Top Row"=w334, "Value"=w334, "Item Symbols"=w335) -> ()  [unwired: 2 in, 2 out]
          }
        }
      }
      event "Listbox": Key Down {
        n213 = event-data() -> ("VKey"=w340:T9)  [unwired: 1 in]
        n214 = case shown="\"Left\", \"Right\"" w340 {
          selector: w340 -> [w345 _]
          tunnel: eventvkey."Left" ("VKey") -> [w343 _]
          frame "Left", "Right" {
            n215 = Equal?(x=w343, y=w345) -> (x = y?=w344:bool)
            n216 = Select(t=0, s=w344, f=1) -> (s? t:f=w346:i32)
            n217 = property on="Listbox" class="LstBox (strict)"() -> ("Item Symbols"=w349:i32[])  [unwired: 2 in, 2 out]
            n218 = Replace Array Subset(array=w349, new element=w346, index="Listbox") -> (w348:i32[])
            n219 = property on="Listbox" class="LstBox (strict)"("Item Symbols"=w348) -> ()  [unwired: 2 in, 2 out]
          }
          frame Default {
          }
        }
      }
      event "DB Camera Config": Value Change {
        n220 = event-data() -> ("NewVal"=w353:bool)  [unwired: 1 in]
        n221 = case shown="False" w353 {
          tunnel: w352 -> [w362 _]
          tunnel: [w355 w373] -> w351
          tunnel: w350 -> [w354 w373]
          frame False {
            w369 = "Camera"
            w372 = FALSE ("Visible")
            n222 = local read "Camera Settings"() -> (w361:T3)
            n223 = Index Array(array=w362) -> (element=w365:cluster{string[]})  [unwired: 1 in]
            n224 = Unbundle(w361) -> ("Frame Rate"=w360:i32, "Compression"=w359:i32, "Size"=w363:u16)
            n225 = Unbundle(w365) -> (w364:string[])
            n226 = Index Array(array=w364, index=w363) -> (element=w358:string)
            n227 = call-poly <vilib>:"Write Key.vi"("section"=w369, "value"=w358, "key"="Size", "refnum"=w354) -> ("refnum out"=w371:T8)  [unwired: 2 in, 5 out]
            n228 = call-poly <vilib>:"Write Key.vi"("section"=w369, "value"=w360, "key"="FrameRate", "refnum"=w371) -> ("refnum out"=w370:T8)  [unwired: 1 in, 6 out]
            n229 = property on="Camera Settings" class="Clust (strict)"("Visible"=w372) -> ()  [unwired: 2 in, 2 out]
            n230 = local write "DB Camera Config"(w372) -> ()
            n231 = call-poly <vilib>:"Write Key.vi"("section"=w369, "value"=w359, "key"="Compression", "refnum"=w370) -> ("refnum out"=w356:T8)  [unwired: 1 in, 6 out]
            n232 = call <vilib>:"Close Config Data.vi"("refnum"=w356) -> ("file path"=w357:path)  [unwired: 2 in, 8 out]
            n233 = call <vilib>:"Open Config Data.vi"("configuration file path"=w357) -> ("refnum"=w355:T8)  [unwired: 8 in, 2 out]
          }
          frame True {
            n234 = property on="Camera Settings" class="Clust (strict)"("Visible"=TRUE) -> ()  [unwired: 2 in, 2 out]
          }
        }
      }
      event "Camera Settings": Value Change {
        n235 = event-data() -> ("NewVal"=w386:T3)  [unwired: 1 in]
        n236 = Index Array(array=w382) -> (element=w381:cluster{string[]})  [unwired: 1 in]
        n237 = Unbundle(w386) -> ("Frame Rate"=w377:i32, "Compression"=w376:i32, "Size"=w379:u16)
        n238 = Unbundle(w381) -> (w380:string[])
        n239 = Index Array(array=w380, index=w379) -> (element=w378:string)
        n240 = Format Into String(format string="%s   %dfps   %d%%", w378, w377, w376) -> (resulting string=w383:string)  [unwired: 2 in, 1 out]
        n241 = Build Array(w383) -> (w384:string[])
        n242 = property on="DB Camera Config" class="Bool (strict)"("Strings [4]"=w384) -> ()  [unwired: 2 in, 2 out]
      }
      event "Motor.Enable": Value Change {
        n243 = event-data() -> ("NewVal"=w392:bool)  [unwired: 1 in]
        n244 = Unbundle("Motor") -> ("Value"=w391:dbl)  [unwired: 1 out]
        n245 = Select(t=w391, s=w392, f=0.0) -> (s? t:f=w389:dbl)
        n246 = call <vilib>:"NT Write Number.vi"("Numeric"=w389, "Name"=w388) -> ()  [unwired: 9 in, 1 out]
      }
      event "Slider": Value Change {
        n247 = event-data() -> ("NewVal"=w395:dbl)  [unwired: 1 in]
        n248 = call <vilib>:"NT Write Number.vi"("Numeric"=w395, "Name"=w396) -> ()  [unwired: 9 in, 1 out]
      }
      event "On/Off": Value Change {
        n249 = event-data() -> ("NewVal"=w400:bool)  [unwired: 1 in]
        n250 = Boolean To (0,1)(Boolean=w400) -> (0, 1=w399:i16)
        n251 = call <vilib>:"NT Write Number.vi"("Numeric"=w399, "Name"=w398) -> ()  [unwired: 9 in, 1 out]
      }
      event "Rev/Fwd": Value Change {
        n252 = event-data() -> ("NewVal.Forward"=w408:bool, "NewVal.Reverse"=w407:bool)  [unwired: 1 in]
        n253 = Boolean To (0,1)(Boolean=w408) -> (0, 1=w404:i16)
        n254 = Boolean To (0,1)(Boolean=w407) -> (0, 1=w406:i16)
        n255 = Negate(x=w406) -> (-x=w405:i16)
        n256 = Add(x=w404, y=w405) -> (x+y=w403:i16)
        n257 = call <vilib>:"NT Write Number.vi"("Numeric"=w403, "Name"=w402) -> ()  [unwired: 9 in, 1 out]
      }
      event "Ring": Value Change {
        n258 = event-data() -> ("NewVal"=w412:u16)  [unwired: 1 in]
        n259 = property on="Ring" class="Ring (strict)"() -> ("Strings []"=w413:string[])  [unwired: 2 in, 2 out]
        n260 = Index Array(array=w413, index=w412) -> (element=w411:string)
        n261 = call <vilib>:"NT Write String.vi"("String"=w411, "Name"=w410) -> ()  [unwired: 9 in, 1 out]
      }
    }
  }
  n262 = Index Array(array=w17) -> (element=w18:cluster{string[]})  [unwired: 1 in]
  n263 = Unbundle(w18) -> (w16:string[])
  n264 = Match First String(2:w16, 3:w15) -> (0:w14:i32)  [unwired: 1 out]
  n265 = Bundle("value"=w20, "value"=w19, "index"=w14) -> (w8:cluster{"value":i32, "value":i32, "index":i32})  [unwired: 1 out]
  n266 = property on="On/Off" class="Bool (strict)"("Visible"=w31) -> ()  [unwired: 2 in, 2 out]
  n267 = property on="Motor" class="Clust (strict)"("Visible"=w31) -> ()  [unwired: 2 in, 2 out]
  n268 = property on="Camera Settings" class="Clust (strict)"("Val(Sgnl)"=w8) -> ()  [unwired: 2 in, 2 out]
  n269 = property on="Rev/Fwd" class="Clust (strict)"("Visible"=w31) -> ()  [unwired: 2 in, 2 out]
  n270 = property on="Progress" class="Clust (strict)"("Visible"=w31) -> ()  [unwired: 2 in, 2 out]
  n271 = property on="Camera Settings" class="Clust (strict)"("Visible"=w31) -> ()  [unwired: 2 in, 2 out]
  n272 = local write "DB Camera Config"(w31) -> ()
  n273 = property on="Ring" class="Ring (strict)"("Visible"=w31) -> ()  [unwired: 2 in, 2 out]
